vi "TH260_CalcBinningValues.vi"(10 "BaseRes":dbl=1.0, 11 "Bin Steps":i32) -> (3 "BinningValues":cluster{"String":string, "Value":i32}[](array[cluster]))   [LabVIEW 2017]
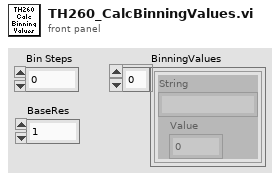
[diagram p1: front panel]
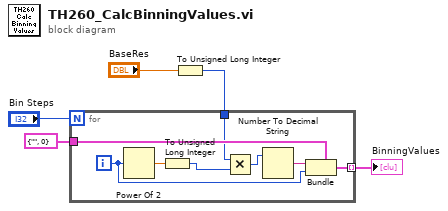
[diagram p0: block diagram]
diagram:
  n1 = To Unsigned Long Integer(number="BaseRes") -> (unsigned 32bit integer=w1:u32)
  n2 = for {
    N: "Bin Steps" -> [_]
    tunnel: cluster{"String":string, "Value":i32} {"String"="", "Value"=0} -> [w13]
    tunnel: [w7] -> w5 mode=indexing
    tunnel: w1 -> [w6]
    i -> [w12]
    n3 = Power Of 2(x=w12) -> (2^x=w11:dbl)
    n4 = To Unsigned Long Integer(number=w11) -> (unsigned 32bit integer=w10:u32)
    n5 = Multiply(x=w6, y=w10) -> (x*y=w9:u32)
    n6 = Number To Decimal String(number=w9) -> (decimal integer string=w8:string)  [unwired: 1 in]
    n7 = Bundle(cluster=w13, "String"=w8, "Value"=w12) -> (w7:cluster{"String":string, "Value":i32})
  }
  "BinningValues" <- w5
